vi "Get Errors.vi"(8 "error in (no error)":errorcluster, 10 "Parse All":bool, 11 "Plugin Manager in":refnum<class "CIFPluginManager.lvclass">) -> (0 "error out":errorcluster, 2 "Errors":T1[](array[typedef]), 3 "Plugin Manager out":refnum<class "CIFPluginManager.lvclass">)   [LabVIEW 2021, in "CIFPluginManager.lvclass"]
uses:
  CIFPluginManager.lvclass
  CIFUtilities/CIFLogs/Typedef/Error Message.ctl
  CIFPluginManager.lvclass/CIFPluginManager.ctl
  CIFUtilities/CIFLogs/CIFLogs.lvlib
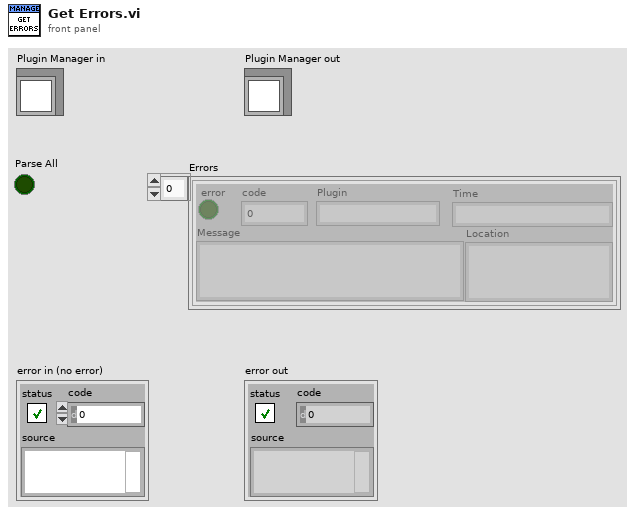
[diagram p1: front panel]
types:
  T1 = typedef "CIFLogs.lvlib/Error Message.ctl" = cluster{"error":bool, "code":i32, "Message":string, "Location":string, "Plugin":string, "Time":string}
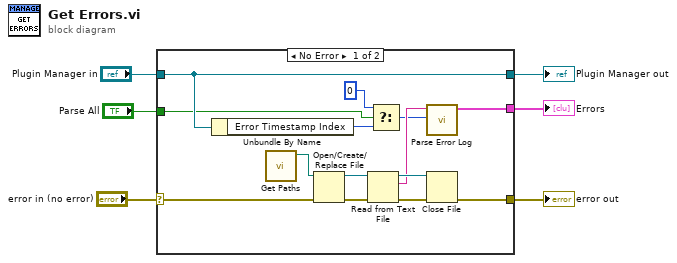
[diagram p0: block diagram]
diagram:
  n1 = case shown="No Error" "error in (no error)" {
    selector: "error in (no error)" -> [w18 w22]
    tunnel: [w15 w22] -> w5
    tunnel: [w12 w21] -> w3
    tunnel: "Plugin Manager in" -> [w12 w21]
    tunnel: [w11 _] -> w2
    tunnel: "Parse All" -> [w7 _]
    frame No Error {
      n2 = Unbundle By Name(w12) -> ("Error Timestamp Index"=w10:u64)
      n3 = call "Get Paths.vi"() -> ("Error Log"=w14:path)  [unwired: 9 in, 2 out]
      n4 = Open/Create/Replace File(file path (use dialog)=w14, error in=w18) -> (refnum out=w19:refnum<file>, error out=w17:errorcluster)  [unwired: 4 in, 1 out]
      n5 = Read from Text File(file (use dialog)=w19, error in=w17) -> (refnum out=w20:refnum<file>, text=w13:string, error out=w16:errorcluster)  [unwired: 2 in, 1 out]
      n6 = Select(t=u64 0, s=w7, f=w10) -> (s? t:f=w9:u64)
      n7 = call "Parse Error Log.vi"("Index Timestamp"=w9, "Error Log"=w13) -> ("Errors"=w11:T1[])  [unwired: 9 in]
      n8 = Close File(refnum=w20, error in=w16) -> (error out=w15:errorcluster)  [unwired: 1 out]
    }
    frame Error {
    }
  }
  "error out" <- w5
  "Plugin Manager out" <- w3
  "Errors" <- w2
